vi "GetEvents.vi"(8 "error in (no error)":errorcluster, 11 "Camera in":refnum<class "CameraI2COUSB.lvclass">) -> (0 "error out":errorcluster, 2 "CameraEvents":T1, 3 "Camera out":refnum<class "CameraI2COUSB.lvclass">)   [LabVIEW 2020, in "CameraI2COUSB.lvlib" / "CameraI2COUSB.lvclass"]
doc: "Return events generates from camera"
uses:
  CameraI2COUSB.lvclass
  ICamera/TypeDef/Events.ctl
  ICamera/TypeDef/StreamDataEvent.ctl
  CameraI2COUSB.lvclass/CameraI2COUSB.ctl
  ICamera/TypeDef/ICamera_typedef.lvlib
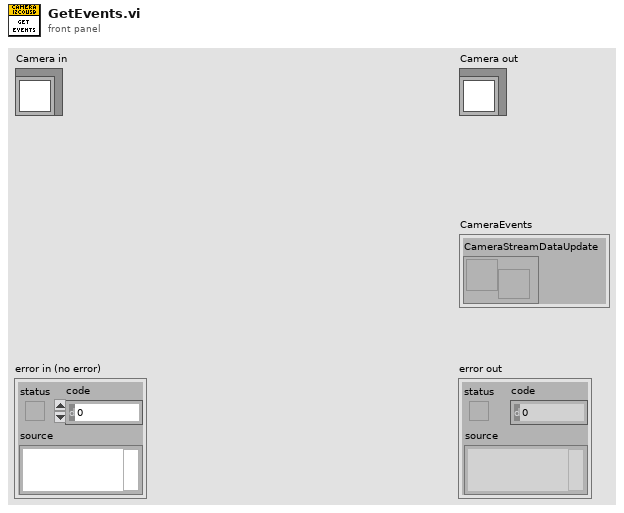
[diagram p1: front panel]
types:
  T1 = typedef "ICamera_typedef.lvlib/Events.ctl" = cluster{"CameraStreamDataUpdate":T2}
  T2 = typedef "ICamera_typedef.lvlib/StreamDataEvent.ctl" = refnum<user-event>
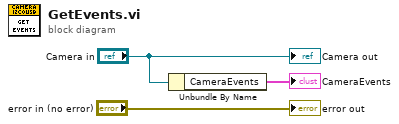
[diagram p0: block diagram]
diagram:
  n1 = Unbundle By Name("Camera in") -> ("CameraEvents"=→"CameraEvents":T1)
  "error out" <- "error in (no error)"
  "Camera out" <- "Camera in"
